vi "AngleDistanceCalc.vi"(8 "Target Angle":dbl, 11 "Current Angle":dbl) -> (0 "Invert drive":bool, 2 "Angle Distance":dbl)   [LabVIEW 2016]
uses:
  Robot Global Data.vi
panel:
  out "angle":dbl
  out "inverted angle":dbl
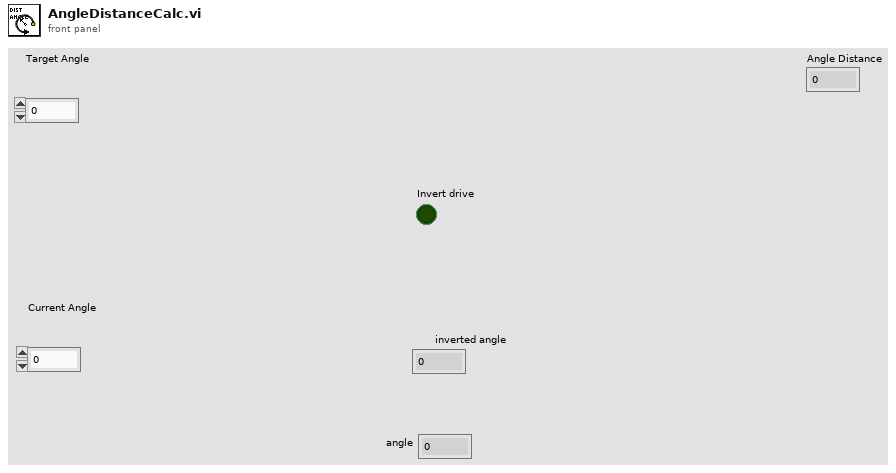
[diagram p1: front panel]
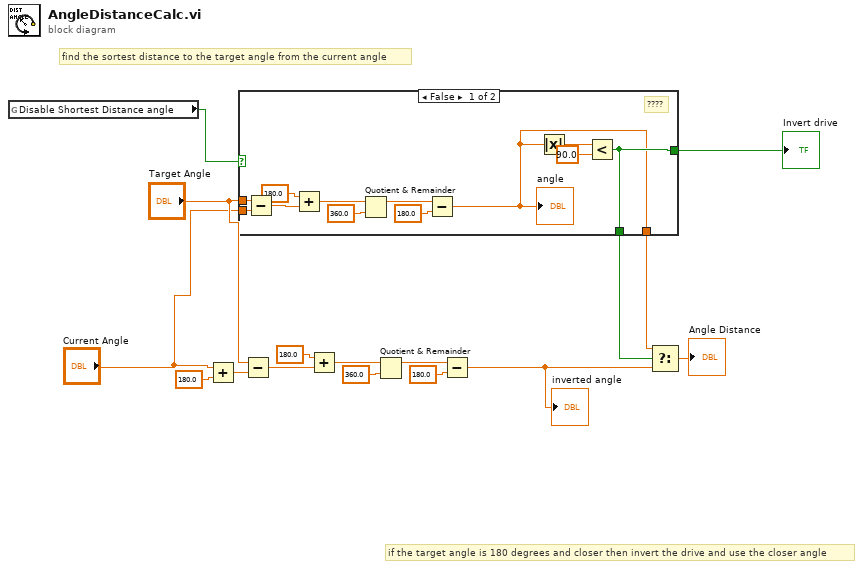
[diagram p0: block diagram]
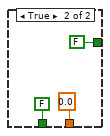
[diagram p2: hidden frame]
diagram:
  # "if the target angle is 180 degrees and closer then invert the drive and use the closer angle"
  # "find the sortest distance to the target angle from the current angle"
  n1 = global read "Robot Global Data.vi" "Disable Shortest Distance angle"() -> (w1:bool)
  n2 = Add(x="Current Angle", y=180.0) -> (x+y=w7:dbl)
  n3 = case shown="False" w1 {
    tunnel: "Target Angle" -> [w27 _]
    tunnel: "Current Angle" -> [w26 _]
    tunnel: [w25 0.0] -> w3
    tunnel: [w16 FALSE] -> w2
    tunnel: [w16 FALSE] -> _
    frame False {
      # "????"
      n4 = Subtract(x=w27, y=w26) -> (x-y=w20:dbl)
      n5 = Add(x=180.0, y=w20) -> (x+y=w19:dbl)
      n6 = Quotient & Remainder(x=w19, y=360.0) -> (x-y*floor(x/y)=w21:dbl)  [unwired: 1 out]
      n7 = Subtract(x=w21, y=180.0) -> (x-y=w25:dbl)
      "angle" <- w25
      n8 = Absolute Value(x=w25) -> (abs(x)=w18:dbl)
      n9 = Less?(x=w18, y=90.0) -> (x < y?=w16:bool)
    }
    frame True {
    }
  }
  "Invert drive" <- w2
  n10 = Subtract(x="Target Angle", y=w7) -> (x-y=w11:dbl)
  n11 = Add(x=180.0, y=w11) -> (x+y=w10:dbl)
  n12 = Quotient & Remainder(x=w10, y=360.0) -> (x-y*floor(x/y)=w12:dbl)  [unwired: 1 out]
  n13 = Subtract(x=w12, y=180.0) -> (x-y=w5:dbl)
  "inverted angle" <- w5
  n14 = Select(t=w3, s=w2, f=w5) -> (s? t:f=→"Angle Distance":dbl)
